vi "button that only gives you true.vi"() -> ()   [LabVIEW 2021]
panel:
  in  "stop":bool
  out "Boolean":bool
  in  "OK Button":bool
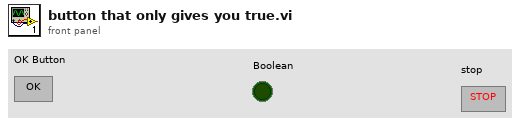
[diagram p1: front panel]
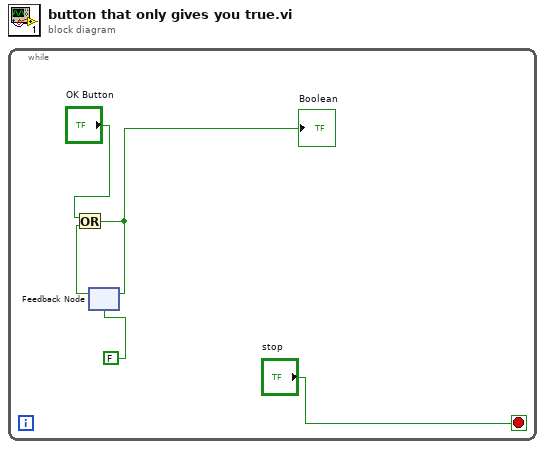
[diagram p0: block diagram]
diagram:
  n1 = while {
    stop <- "stop" stop-if-true
    n2 = feedback #1(FALSE) -> (w4:bool)
    n3 = Or(x="OK Button", y=w4) -> (x .or. y?=w2:bool)
    "Boolean" <- w2
    n4 = feedback-in #1(w2) -> ()
  }
